vi "ProcessState-Starting.vi"(2 "PROCESS":string, 9 "error in (no error)":errorcluster) -> (0 "ProcessStateNotifier":refnum<notifier>, 6 "error in (no error)":errorcluster caption="error out")   [LabVIEW 2009]
uses:
  ProcessState.ctl
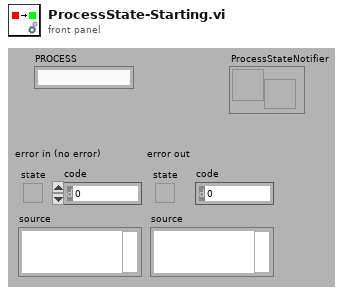
[diagram p1: front panel]
types:
  T1 = typedef "ProcessState.ctl" = enum16{"STARTING", "RUNNING", "STOPPING", "STOPPPED"}
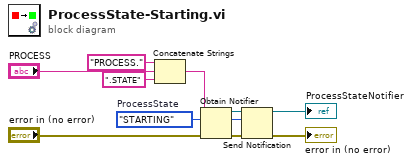
[diagram p0: block diagram]
diagram:
  w3 = ProcessState."STARTING"  # ProcessState
  n1 = Concatenate Strings("PROCESS." ("chaîne"), "PROCESS", ".STATE" ("chaîne")) -> (w7:string)
  n2 = Obtain Notifier(name (unnamed)=w7, notification data type=w3, error in (no error)="error in (no error)") -> (notifier out=w4:refnum<notifier>, error out=w5:errorcluster)  [unwired: 1 in, 1 out]
  n3 = Send Notification(notification=w3, notifier=w4, error in (no error)=w5) -> (notifier out=→"ProcessStateNotifier":refnum<notifier>, error out=→"error in (no error)":errorcluster)
